vi "Main_20a.vi"() -> ()   [LabVIEW 2023]
uses:
  ENUM_Type.ctl
  Cluster_Part.ctl
panel:
  in  "Example 2":string="broadcaster -> a\n%a -> inv, con\n&inv -> b\n%b -> con\n&con -> output"
  out "Answer":u32
  in  "Puzzle":string="%cf -> hl, qt\n&bn -> rx\n%nb -> vt\n%hm -> jp\n%vr -> qt, sl\n%gq -> hm, nl\n%sl -> jx, qt\n&pl -> bn\n%hf -> vt, ch\n%kx -> dq\n%fr -> qf\n%rh -> vr\n&vt -> lz, dh, kr, kq, lm, qk\n&dq -> mz, ml, xd, fb, xs, rc, rt\n%hn -> qk, vt\n%bv -> nl\n%jv -> rh, qt\n%kq -> lm\n%nd -> hp\n%gj -> bv, nl\n%lv -> xs, dq\n%ch -> vt, kd\n%sm -> qt, nd\n%nt -> jv\n%qk -> cb\n%jx -> cf\n%hl -> qt, ng\n&qt -> sm, rh, nd, jx, nt, pl\n%bh -> nl, fr\n%kd -> vt, nb\n%gx -> mh, dq\n%hp -> nt, qt\n%rc -> lv\nbroadcaster -> kr, zb, sm, xd\n&mz -> bn\n%qf -> rd, nl\n%sk -> nl, bh\n%rb -> nl, sk\n%cb -> hf, vt\n%fb -> rt\n&lz -> bn\n%mh -> dq, kx\n%rt -> mt\n%xd -> dq, fb\n%lm -> hn\n%hh -> vt, dh\n%ml -> ts\n%mt -> rc, dq\n%ts -> gx, dq\n%rd -> nl, gq\n%zb -> nl, rb\n%kr -> hh, vt\n&nl -> fr, zb, hm, zm\n&zm -> bn\n%dh -> kq\n%ng -> qt\n%xs -> ml\n%jp -> nl, gj"
  in  "Example":string="broadcaster -> a, b, c\n%a -> b\n%b -> c\n%c -> inv\n&inv -> a"
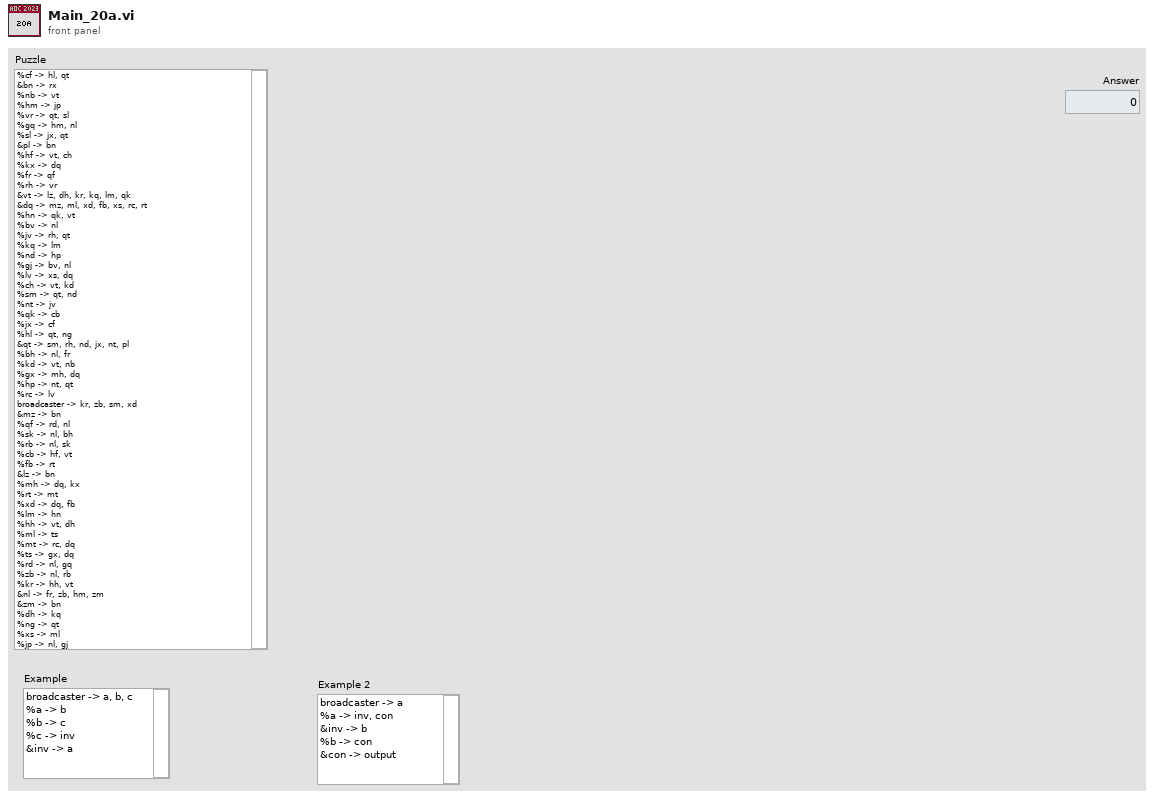
[diagram p1: front panel]
types:
  T1 = typedef "ENUM_Type.ctl" = enum16{"Start Button", "Broadcaster", "FlipFlop", "Conjuction"}
  T2 = typedef "Cluster_Part.ctl" = cluster{"Type":T1, "Outputs":string[]}
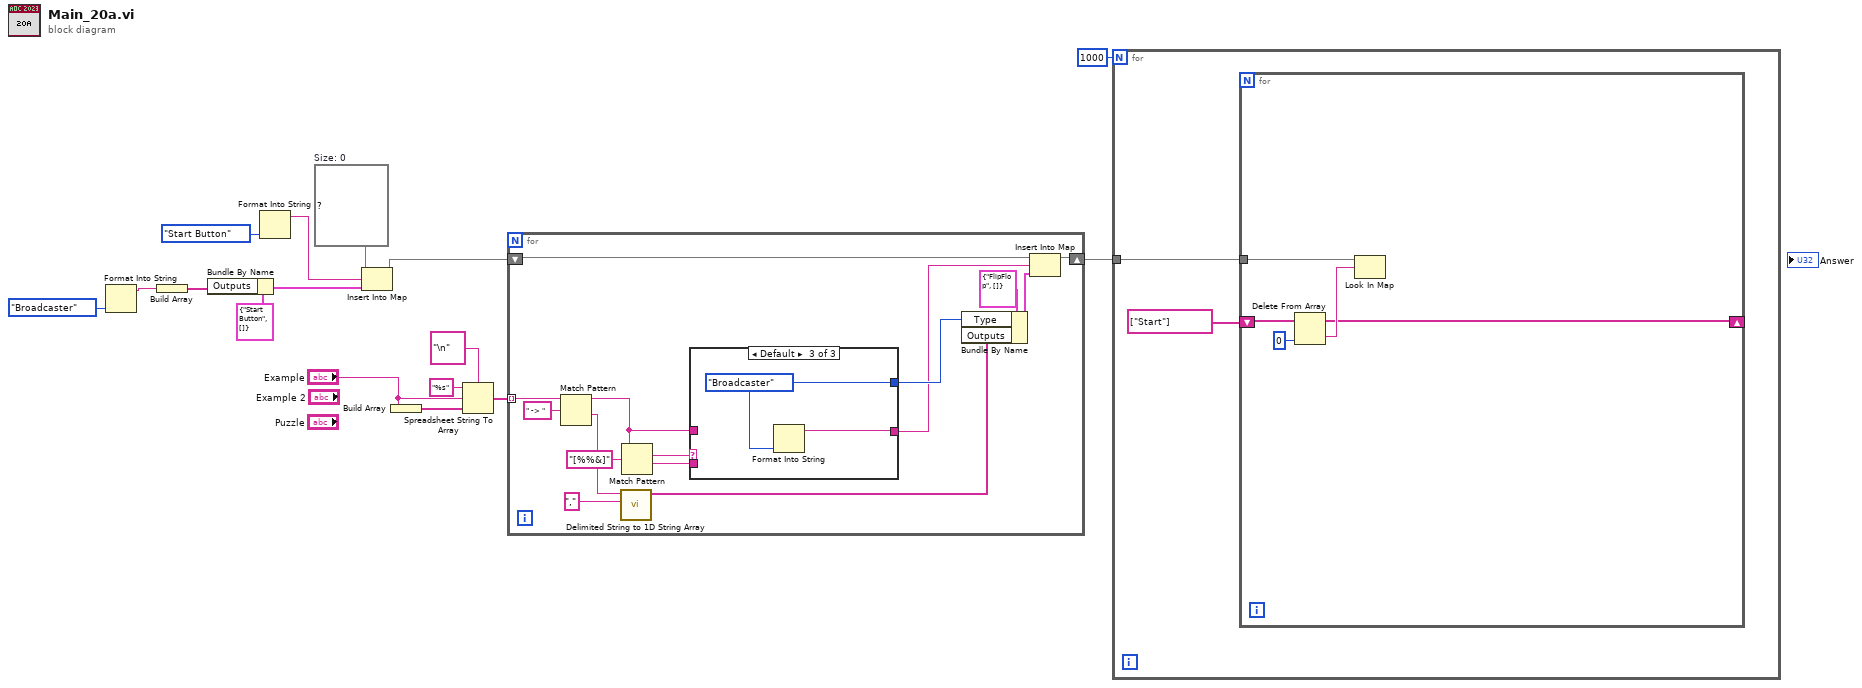
[diagram p0: block diagram]
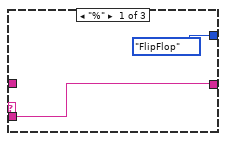
[diagram p2: hidden frame]
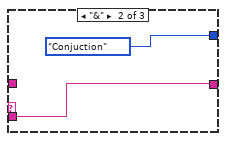
[diagram p3: hidden frame]
diagram:
  w11 = map{string, T2} {}  # Size: 0
  n1 = Format Into String(ENUM_Type."Broadcaster" ("Enum")) -> (resulting string=w8:string)  [unwired: 3 in, 1 out]
  n2 = Build Array(w8) -> (w6:string[])
  n3 = Bundle By Name(cluster=T2 {"Type"=enum."Start Button", "Outputs"=[]} ("value"), "Outputs"=w6) -> (w7:T2)
  n4 = Format Into String(ENUM_Type."Start Button" ("Enum")) -> (resulting string=w3:string)  [unwired: 3 in, 1 out]
  n5 = Insert Into Map(map in=w11, key=w3, value=w7) -> (map out=w10:map{string, T2})  [unwired: 2 out]
  n6 = Build Array("Example") -> (w16:string[])
  n7 = Spreadsheet String To Array(delimiter (Tab)="\n", format string="%s", spreadsheet string="Example", array type (2D Dbl)=w16) -> (array=w12:string[])
  n8 = for {
    tunnel: w12 -> [w31] mode=indexing
    shift-right: [w19] -> w2
    shift-left: w10 -> [w20]
    n9 = Match Pattern(string=w31, regular expression=" -> ") -> (before substring=w25:string, after substring=w24:string)  [unwired: 1 in, 2 out]
    n10 = call <vilib>:"Delimited String to 1D String Array.vi"("delimiter"=",", "delimited string"=w24) -> ("string array"=w21:string[])  [unwired: 9 in]
    n11 = Match Pattern(string=w25, regular expression="[%%&]") -> (match substring=w27:string, after substring=w26:string)  [unwired: 1 in, 2 out]
    n12 = case shown="Default" w27 {
      tunnel: w26 -> [w33 w35 _]
      tunnel: w25 -> [_ _ _]
      tunnel: [w33 w35 w36] -> w18
      tunnel: [ENUM_Type."FlipFlop" ("Enum") ENUM_Type."Conjuction" ("Enum") w37] -> w22
      frame "%" {
      }
      frame "&" {
      }
      frame Default {
        w37 = ENUM_Type."Broadcaster" ("Enum")
        n13 = Format Into String(w37) -> (resulting string=w36:string)  [unwired: 3 in, 1 out]
      }
    }
    n14 = Bundle By Name(cluster=T2 {"Type"=enum."FlipFlop", "Outputs"=[]}, "Type"=w22, "Outputs"=w21) -> (w17:T2)
    n15 = Insert Into Map(map in=w20, key=w18, value=w17) -> (map out=w19:map{string, T2})  [unwired: 2 out]
  }
  n16 = for {
    N: 1000 -> [_]
    tunnel: w2 -> [w39]
    n17 = for {
      shift-right: [w40] -> _
      shift-left: string[] ["Start"] -> [w44]
      tunnel: w39 -> [w42]
      n18 = Delete From Array(array=w44, index=0) -> (deleted portion=w41:string, array with subset deleted=w40:string[])  [unwired: 1 in]
      n19 = Look In Map(map=w42, key=w41) -> ()  [unwired: 1 in, 2 out]
    }
  }
